vi "stage_move_relative.vi"(7 "Stage Name":string, 8 "error in (no error)":errorcluster, 9 "wait_for_done":bool, 10 "increment":dbl, 11 "newport_xps in":refnum<class "newport_xps.lvclass">) -> (0 "error out":errorcluster, 3 "newport_xps out":refnum<class "newport_xps.lvclass">)   [LabVIEW 2015, in "newport_xps.lvclass"]
uses:
  newport_xps.lvclass
  newport_xps.lvclass/newport_xps.ctl
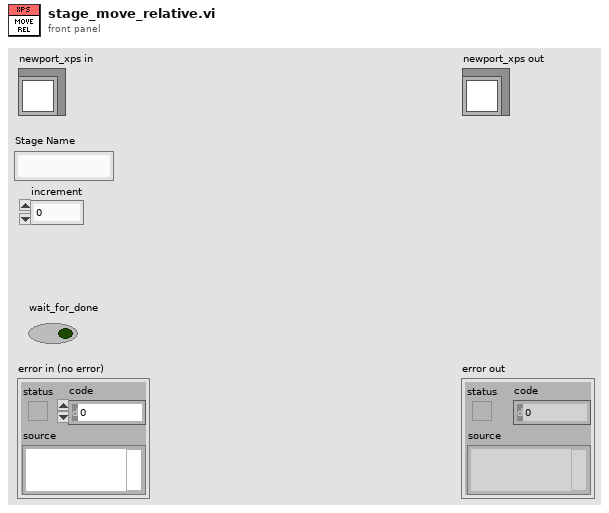
[diagram p1: front panel]
types:
  T1 = cluster{"connection TCP":refnum<k5>, "LogTo File":bool, "Log File refnum":refnum<file>, "no error if error log":bool}
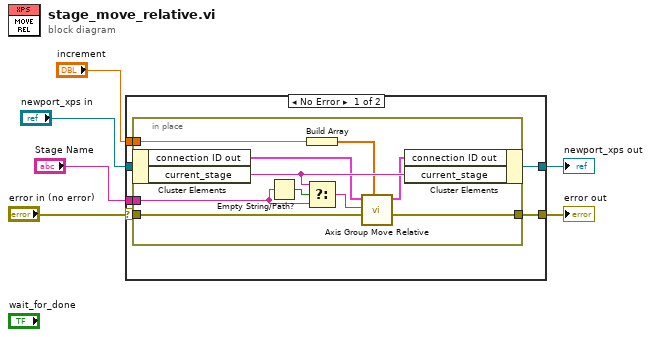
[diagram p0: block diagram]
diagram:
  n1 = case shown="No Error" "error in (no error)" {
    selector: "error in (no error)" -> [w10 w24]
    tunnel: "newport_xps in" -> [w12 w23]
    tunnel: "Stage Name" -> [w11 _]
    tunnel: "increment" -> [w9 _]
    tunnel: [w8 w24] -> w2
    tunnel: [w7 w23] -> w1
    frame No Error {
      n2 = in-place {
        in-place-border: w11 -> [w20]
        in-place-border: w10 -> [w18]
        in-place-border: w9 -> [w22]
        in-place-border: [w17] -> w8
        n3 = in-place-cluster #1(w12) -> ("connection ID out"=w16:T1, "current_stage"=w19:string)
        n4 = Empty String/Path?(string/path=w20) -> (empty?=w21:bool)
        n5 = Build Array(w22) -> (w14:dbl[])
        n6 = Select(t=w19, s=w21, f=w20) -> (s? t:f=w13:string)
        n7 = call "Axis Group Move Relative.vi"("Target Displacement (units)"=w14, "XPS error in (no error)"=w18, "Group Name (250 c max)"=w13, "connection ID in"=w16) -> ("XPS error out"=w17:errorcluster, "connection ID out"=w15:T1)  [unwired: 5 in, 1 out]
        n8 = in-place-cluster #1("connection ID out"=w15, "current_stage"=w19) -> (w7:refnum<class "newport_xps.lvclass">)
      }
    }
    frame Error {
    }
  }
  "error out" <- w2
  "newport_xps out" <- w1
